vi "Medição_temperaturas.vi"() -> ()   [LabVIEW 2018]
uses:
  <vilib>/Utility/file.llb/Write Delimited Spreadsheet (DBL).vi
panel:
  out "String":string
  in  "Nome do arquivo (p, U, pos, i)":string="default"
  out "Waveform Graph":dbl[][](graph)
  out "T sala":dbl
  in  "STOP":bool
  out "T2":dbl
  out "T1":dbl
  out "T0":dbl
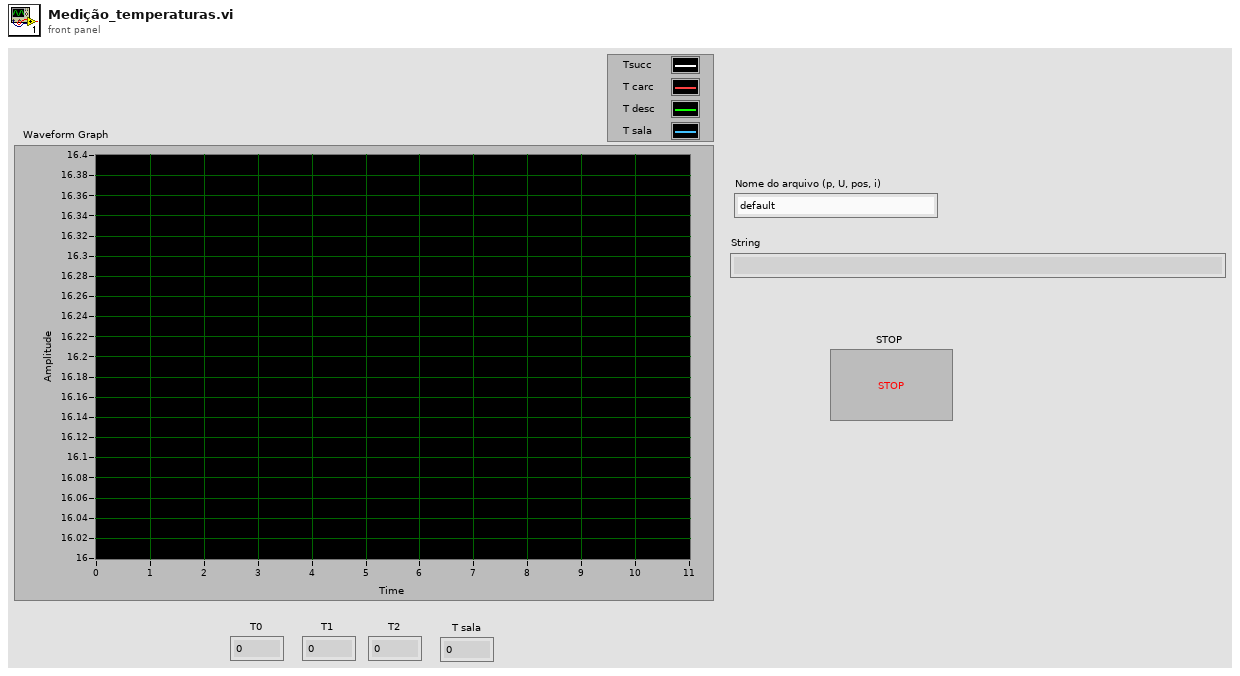
[diagram p1: front panel]
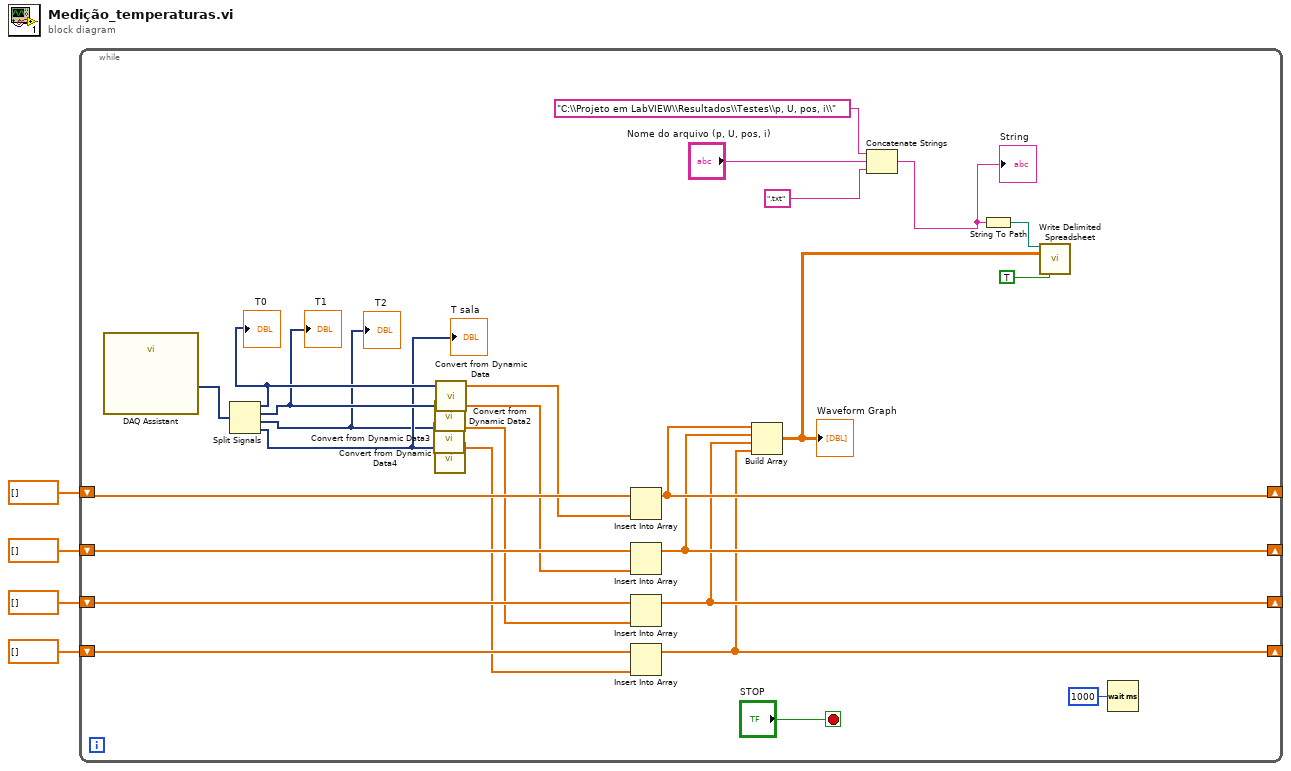
[diagram p0: block diagram]
diagram:
  n1 = while {
    shift-right: [w16] -> _
    shift-left: dbl[] [] -> [w24]
    shift-right: [w15] -> _
    shift-left: dbl[] [] -> [w23]
    shift-right: [w14] -> _
    shift-left: dbl[] [] -> [w22]
    shift-right: [w13] -> _
    shift-left: dbl[] [] -> [w21]
    stop <- "STOP" stop-if-true
    n2 = call "DAQ Assistant"() -> ("data"=w30:dynamicdata)  [unwired: 17 in, 2 out]
    n3 = Split Signals(w30) -> (w28:dynamicdata, w27:dynamicdata, w25:dynamicdata, w26:dynamicdata)  [unwired: 4 in]
    "T0" <- w28
    "T1" <- w27
    "T2" <- w25
    "T sala" <- w26
    n4 = call "Convert from Dynamic Data3"("Dynamic Data Type"=w25) -> ("Array"=w18:dbl[])  [unwired: 3 in]
    n5 = call "Convert from Dynamic Data2"("Dynamic Data Type"=w27) -> ("Array"=w19:dbl[])  [unwired: 3 in]
    n6 = call "Convert from Dynamic Data4"("Dynamic Data Type"=w26) -> ("Array"=w17:dbl[])  [unwired: 3 in]
    n7 = call "Convert from Dynamic Data"("Dynamic Data Type"=w28) -> ("Array"=w20:dbl[])  [unwired: 3 in]
    n8 = Insert Into Array(array=w24, new element=w20) -> (w16:dbl[])  [unwired: 1 in]
    n9 = Insert Into Array(array=w23, new element=w19) -> (w15:dbl[])  [unwired: 1 in]
    n10 = Insert Into Array(array=w22, new element=w18) -> (w14:dbl[])  [unwired: 1 in]
    n11 = Insert Into Array(array=w21, new element=w17) -> (w13:dbl[])  [unwired: 1 in]
    n12 = Build Array(w16, w15, w14, w13) -> (w6:dbl[][])
    "Waveform Graph" <- w6
    n13 = Concatenate Strings("C:\\Projeto em LabVIEW\\Resultados\\Testes\\p, U, pos, i\\", "Nome do arquivo (p, U, pos, i)", ".txt") -> (w10:string)
    "String" <- w10
    n14 = String To Path(string=w10) -> (path=w7:path)
    n15 = call-poly <vilib>:"Write Delimited Spreadsheet.vi"("file path (dialog if empty)"=w7, "2D data"=w6, "transpose? (no:F)"=TRUE) -> ()  [unwired: 11 in, 2 out]
    n16 = Wait (ms)(milliseconds to wait=u32 1000) -> ()  [unwired: 1 out]
  }
